vi "Main.vi"() -> ()   [LabVIEW 2019]
uses:
  <vilib>/Native 3D Graph/xcontrol/3DPC_SurfacePlot.xctl
  <vilib>/Analysis/coordinate.llb/3D Coordinate Conversion (Array).vi
  <vilib>/Analysis/_algsub.llb/Real Vector Norm.vi
  <vilib>/Utility/file.llb/Read Delimited Spreadsheet (DBL).vi
  <vilib>/Analysis/polynomials.llb/Polynomial Roots (DBL).vi
  <vilib>/Analysis/NI_AALPro.lvlib
  <vilib>/Analysis/NI_AAL_Geometry.lvlib
panel:
  out "chegada":dbl[](array[numeric])
  out "partida":dbl[](array[numeric])
  out "Areas dos triangulos":dbl[](array[numeric])
  out "Primeiro":dbl[](array[numeric])
  out "Ultimo":dbl[](array[numeric])
  out "origem z":dbl
  out "origem y":dbl
  out "origem x":dbl
  out "Roots YZ":cdb[](array[numeric])
  out "Roots XZ":cdb[](array[numeric])
  out "3D Graph 2":refnum<class "Base Datatype.lvclass">[](xcontrol)
  out "Right 2":cluster{"Y":dbl[], "Y":dbl[]}[](graph)
  out "Front 2":cluster{"Y":dbl[], "Y":dbl[]}[](graph)
  out "Top 2":cluster{"Y":dbl[], "Y":dbl[]}[](graph)
  out "Right":cluster{"Y":dbl[], "Y":dbl[]}[](graph)
  out "Front":cluster{"Y":dbl[], "Y":dbl[]}[](graph)
  out "Top":cluster{"Y":dbl[], "Y":dbl[]}[](graph)
  out "3D Graph":refnum<class "Base Datatype.lvclass">[](xcontrol)
  # "Localizaçao da origem"
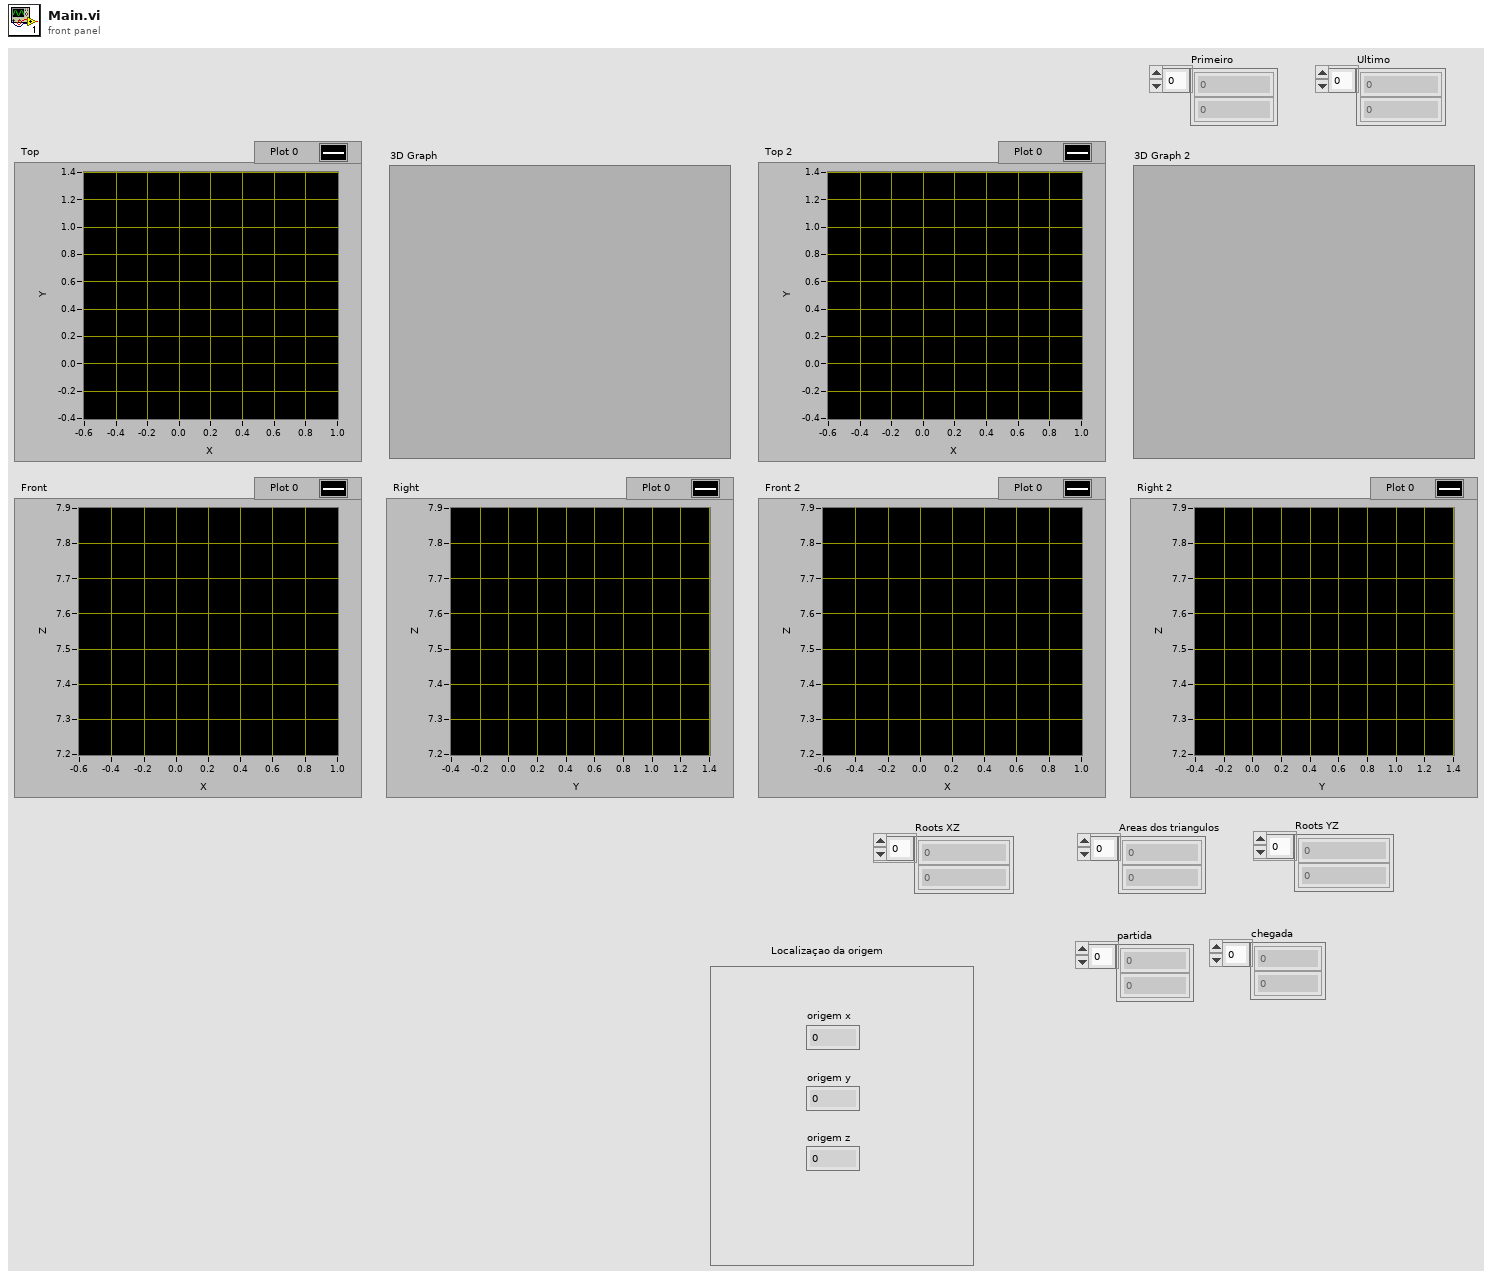
[diagram p1: front panel]
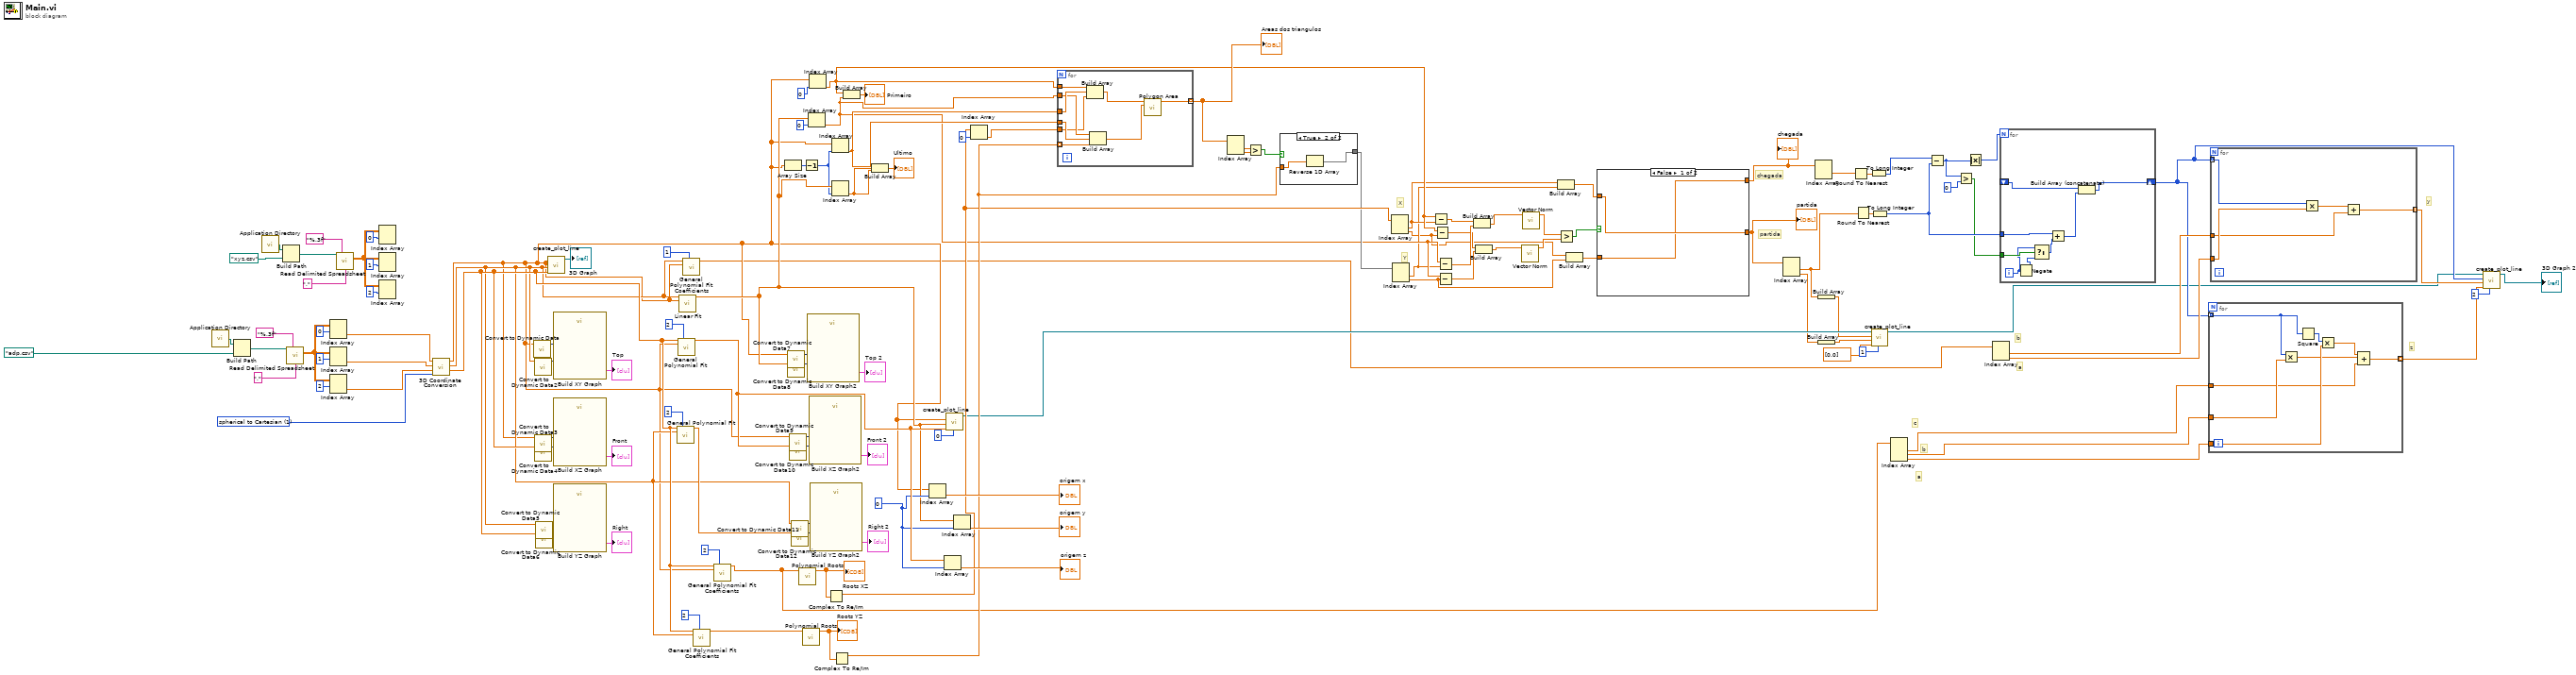
[diagram p0: block diagram]
diagram:
  w73 = 0
  w91 = u16 1 items=["Cartesian to spherical", "spherical to Cartesian", "Cartesian to cylindrical", "cylindrical to Cartesian", "spherical to cylindrical", "cylindrical to spherical"] ("conversion type")
  # "y"
  # "z"
  # "b"
  # "a"
  # "c"
  # "b"
  # "a"
  # "partida"
  # "chegada"
  # "Y"
  # "X"
  n1 = call <vilib>:"Application Directory.vi"() -> ("Application Directory"=w88:path)
  n2 = Build Path(base path=w88, name or relative path=path "adp.csv" ("file path (dialog if empty)")) -> (appended path=w89:path)
  n3 = call <vilib>:"Application Directory.vi"() -> ("Application Directory"=w123:path)
  n4 = Build Path(base path=w123, name or relative path=path "xyz.csv" ("file path (dialog if empty)")) -> (appended path=w124:path)
  n5 = call-poly <vilib>:"Read Delimited Spreadsheet.vi"("file path (dialog if empty)"=w89, "format (%.3f)"="%.3f", "delimiter (\\t)"="," ("delimiter (\\t)")) -> ("all rows"=w82:dbl[][])  [unwired: 7 in, 5 out]
  n6 = Index Array(array=w82, index (row)=0) -> (element=w78:dbl[])  [unwired: 1 in]
  n7 = Index Array(array=w82, index (row)=1) -> (element=w79:dbl[])  [unwired: 1 in]
  n8 = Index Array(array=w82, index (row)=2) -> (element=w80:dbl[])  [unwired: 1 in]
  n9 = call-poly <vilib>:"Read Delimited Spreadsheet.vi"("file path (dialog if empty)"=w124, "format (%.3f)"="%.3f", "delimiter (\\t)"="," ("delimiter (\\t)")) -> ("all rows"=w116:dbl[][])  [unwired: 7 in, 5 out]
  n10 = Index Array(array=w116, index (row)=0) -> ()  [unwired: 1 in, 1 out]
  n11 = Index Array(array=w116, index (row)=1) -> ()  [unwired: 1 in, 1 out]
  n12 = Index Array(array=w116, index (row)=2) -> ()  [unwired: 1 in, 1 out]
  n13 = call-poly <vilib>:"3D Coordinate Conversion.vi"("conversion type"=w91, "Axis 3"=w80, "Axis 2"=w79, "Axis 1"=w78) -> ("Axis 3 Out"=w81:dbl[], "Axis 2 Out"=w14:dbl[], "Axis 1 Out"=w13:dbl[])  [unwired: 4 in, 1 out]
  n14 = call "Convert to Dynamic Data"("Array"=w13) -> ("Dynamic Data Type"=w114:dynamicdata)  [unwired: 3 in]
  n15 = call "Convert to Dynamic Data2"("Array"=w14) -> ("Dynamic Data Type"=w113:dynamicdata)  [unwired: 3 in]
  n16 = call "Convert to Dynamic Data3"("Array"=w13) -> ("Dynamic Data Type"=w110:dynamicdata)  [unwired: 3 in]
  n17 = call "Convert to Dynamic Data4"("Array"=w81) -> ("Dynamic Data Type"=w109:dynamicdata)  [unwired: 3 in]
  n18 = call "Convert to Dynamic Data5"("Array"=w14) -> ("Dynamic Data Type"=w108:dynamicdata)  [unwired: 3 in]
  n19 = call "Convert to Dynamic Data6"("Array"=w81) -> ("Dynamic Data Type"=w107:dynamicdata)  [unwired: 3 in]
  n20 = call <vilib>:"create_plot_line.vi"("z vector"=w81, "y vector"=w14, "x vector"=w13) -> ("plots out"=→"3D Graph":refnum<class "Base Datatype.lvclass">[])  [unwired: 2 in, 6 out]
  n21 = call "Build XY Graph"("Y Input"=w113, "X Input"=w114) -> ("XY Graph"=→"Top":cluster{"X":dbl[], "Y":dbl[]}[])  [unwired: 8 in, 1 out]
  n22 = call "Build XZ Graph"("Y Input"=w109, "X Input"=w110) -> ("XY Graph"=→"Front":cluster{"X":dbl[], "Y":dbl[]}[])  [unwired: 8 in, 1 out]
  n23 = call "Build YZ Graph"("Y Input"=w107, "X Input"=w108) -> ("XY Graph"=→"Right":cluster{"X":dbl[], "Y":dbl[]}[])  [unwired: 8 in, 1 out]
  n24 = call <vilib>:"General Polynomial Fit.vi"("Y"=w81, "polynomial order"=2, "X"=w14) -> ("Best Polynomial Fit"=w95:dbl[])  [unwired: 9 in, 3 out]
  n25 = call <vilib>:"General Polynomial Fit.vi"("Y"=w81, "polynomial order"=2, "X"=w13) -> ("Best Polynomial Fit"=w75:dbl[])  [unwired: 9 in, 3 out]
  n26 = call <vilib>:"Linear Fit.vi"("Y"=w14, "X"=w13) -> ("Best Linear Fit"=w70:dbl[])  [unwired: 9 in, 4 out]
  n27 = call <vilib>:"General Polynomial Fit Coefficients.vi"("Y"=w14, "polynomial order"=1, "X"=w13) -> ("Polynomial Coefficients"=w11:dbl[])  [unwired: 11 in, 1 out]
  n28 = call <vilib>:"General Polynomial Fit Coefficients.vi"("Y"=w81, "polynomial order"=2, "X"=w14) -> ("Polynomial Coefficients"=w92:dbl[])  [unwired: 11 in, 1 out]
  n29 = call <vilib>:"General Polynomial Fit Coefficients.vi"("Y"=w81, "polynomial order"=2, "X"=w13) -> ("Polynomial Coefficients"=w32:dbl[])  [unwired: 11 in, 1 out]
  n30 = Array Size(array=w13) -> (size(s)=w67:i32)
  n31 = call "Convert to Dynamic Data7"("Array"=w13) -> ("Dynamic Data Type"=w105:dynamicdata)  [unwired: 3 in]
  n32 = call "Convert to Dynamic Data8"("Array"=w70) -> ("Dynamic Data Type"=w106:dynamicdata)  [unwired: 3 in]
  n33 = call "Convert to Dynamic Data9"("Array"=w13) -> ("Dynamic Data Type"=w102:dynamicdata)  [unwired: 3 in]
  n34 = call "Convert to Dynamic Data10"("Array"=w75) -> ("Dynamic Data Type"=w103:dynamicdata)  [unwired: 3 in]
  n35 = call "Convert to Dynamic Data11"("Array"=w14) -> ("Dynamic Data Type"=w99:dynamicdata)  [unwired: 3 in]
  n36 = call "Convert to Dynamic Data12"("Array"=w95) -> ("Dynamic Data Type"=w100:dynamicdata)  [unwired: 3 in]
  n37 = call-poly <vilib>:"Polynomial Roots.vi"("P(x)"=w32) -> ("Roots"=w65:cdb[])  [unwired: 9 in, 1 out]
  "Roots XZ" <- w65
  n38 = call-poly <vilib>:"Polynomial Roots.vi"("P(x)"=w92) -> ("Roots"=w64:cdb[])  [unwired: 9 in, 1 out]
  "Roots YZ" <- w64
  n39 = Decrement(x=w67) -> (x-1=w66:i32)
  n40 = call "Build XY Graph2"("Y Input"=w106, "X Input"=w105) -> ("XY Graph"=→"Top 2":cluster{"X":dbl[], "Y":dbl[]}[])  [unwired: 8 in, 1 out]
  n41 = Index Array(array=w70, index=0) -> (element=w51:dbl)
  n42 = Index Array(array=w13, index=0) -> (element=w52:dbl)
  n43 = call "Build XZ Graph2"("Y Input"=w103, "X Input"=w102) -> ("XY Graph"=→"Front 2":cluster{"X":dbl[], "Y":dbl[]}[])  [unwired: 8 in, 1 out]
  n44 = call "Build YZ Graph2"("Y Input"=w100, "X Input"=w99) -> ("XY Graph"=→"Right 2":cluster{"X":dbl[], "Y":dbl[]}[])  [unwired: 8 in, 1 out]
  n45 = Complex To Re/Im(x + iy=w65) -> (x=w54:dbl[])  [unwired: 1 out]
  n46 = Index Array(array=w13, index=w66) -> (element=w63:dbl)
  n47 = Index Array(array=w70, index=w66) -> (element=w62:dbl)
  n48 = Complex To Re/Im(x + iy=w64) -> (x=w55:dbl[])  [unwired: 1 out]
  n49 = Build Array(w52, w51) -> (→"Primeiro":dbl[])
  n50 = Build Array(w63, w62) -> (→"Ultimo":dbl[])
  n51 = Index Array(array=w13, index=w73) -> (element=→"origem x":dbl)
  n52 = Index Array(array=w75, index=w73) -> (element=→"origem z":dbl)
  n53 = call <vilib>:"create_plot_line.vi"("plot ID"=0, "z vector"=w75, "y vector"=w70, "x vector"=w13) -> ("plots out"=w37:refnum<class "Base Datatype.lvclass">[])  [unwired: 1 in, 6 out]
  n54 = Index Array(array=w70, index=w73) -> (element=→"origem y":dbl)
  n55 = Index Array(array=w54, index=0) -> (element=w60:dbl)
  n56 = for {
    tunnel: w55 -> [w130] mode=indexing
    tunnel: w52 -> [w134]
    tunnel: w51 -> [w132]
    tunnel: w63 -> [w133]
    tunnel: w62 -> [w131]
    tunnel: [w127] -> w59 mode=indexing
    tunnel: w60 -> [w126]
    n57 = Build Array(w134, w133, w126) -> (w128:dbl[])
    n58 = Build Array(w132, w131, w130) -> (w129:dbl[])
    n59 = call <vilib>:"Polygon Area.vi"("Y"=w129, "X"=w128) -> ("signed area"=w127:dbl)  [unwired: 8 in, 1 out]
  }
  "Areas dos triangulos" <- w59
  n60 = Index Array(array=w59) -> (element #1=w57:dbl, element #2=w58:dbl)  [unwired: 2 in]
  n61 = Greater?(x=w57, y=w58) -> (0:w56:bool)
  n62 = case shown="True" w56 {
    tunnel: w55 -> [w135 w137]
    tunnel: [w135 w136] -> w53
    frame False {
    }
    frame True {
      n63 = Reverse 1D Array(array=w137) -> (reversed array=w136:dbl[])
    }
  }
  n64 = Index Array(array=w54) -> (element #1=w41:dbl, element #2=w39:dbl)  [unwired: 2 in]
  n65 = Index Array(array=w53) -> (element #1=w40:dbl, element #2=w38:dbl)  [unwired: 2 in]
  n66 = Subtract(x=w52, y=w41) -> (x-y=w50:dbl)
  n67 = Subtract(x=w52, y=w39) -> (x-y=w48:dbl)
  n68 = Subtract(x=w51, y=w40) -> (x-y=w49:dbl)
  n69 = Subtract(x=w51, y=w38) -> (x-y=w47:dbl)
  n70 = Build Array(w50, w49) -> (w43:dbl[])
  n71 = Build Array(w48, w47) -> (w42:dbl[])
  n72 = call-poly <vilib>:"Vector Norm.vi"("Input Vector"=w42) -> ("norm"=w45:dbl)  [unwired: 9 in, 1 out]
  n73 = call-poly <vilib>:"Vector Norm.vi"("Input Vector"=w43) -> ("norm"=w46:dbl)  [unwired: 9 in, 1 out]
  n74 = Build Array(w41, w40) -> (w30:dbl[])
  n75 = Greater?(x=w46, y=w45) -> (0:w44:bool)
  n76 = Build Array(w39, w38) -> (w31:dbl[])
  n77 = case shown="False" w44 {
    tunnel: [w139 w141] -> w29
    tunnel: w31 -> [w138 w141]
    tunnel: w30 -> [w139 w140]
    tunnel: [w138 w140] -> w28
    frame False {
    }
    frame True {
    }
  }
  "partida" <- w29
  "chegada" <- w28
  n78 = Index Array(array=w29) -> (element #1=w26:dbl, element #2=w35:dbl)  [unwired: 2 in]
  n79 = Index Array(array=w28) -> (element #1=w27:dbl)  [unwired: 2 in, 1 out]
  n80 = Build Array(w26) -> (w36:dbl[])
  n81 = Build Array(w35) -> (w34:dbl[])
  n82 = Round To Nearest(number=w27) -> (nearest integer value=w25:dbl)
  n83 = Round To Nearest(number=w26) -> (nearest integer value=w24:dbl)
  n84 = To Long Integer(number=w25) -> (32bit integer=w23:i32)
  n85 = call <vilib>:"create_plot_line.vi"("plot ID"=1, "z vector"=dbl[] [0.0], "y vector"=w34, "x vector"=w36, "plots in"=w37) -> ("plots out"=w5:refnum<class "Base Datatype.lvclass">[])  [unwired: 6 out]
  n86 = To Long Integer(number=w24) -> (32bit integer=w22:i32)
  n87 = Index Array(array=w32) -> (element #1=w15:dbl, element #2=w16:dbl, element #3=w17:dbl)  [unwired: 3 in]
  n88 = Subtract(x=w23, y=w22) -> (x-y=w18:i32)
  n89 = Greater?(x=w18, y=0) -> (0:w19:bool)
  n90 = Absolute Value(x=w18) -> (abs(x)=w21:i32)
  n91 = Index Array(array=w11) -> (element #1=w9:dbl, element #2=w10:dbl)  [unwired: 2 in]
  n92 = for {
    N: w21 -> [_]
    shift-right: [w146] -> w6
    shift-left: _ -> [w149]
    tunnel: w22 -> [w148]
    tunnel: w19 -> [w145]
    i -> [w143]
    n93 = Negate(x=w143) -> (-x=w144:i32)
    n94 = Select(t=w143, s=w145, f=w144) -> (s? t:f=w142:i32)
    n95 = Add(x=w148, y=w142) -> (x+y=w147:i32)
    n96 = Build Array (concatenate)(w149, w147) -> (w146:i32[])
  }
  n97 = for {
    tunnel: w17 -> [w156]
    tunnel: w16 -> [w154]
    tunnel: w15 -> [w151]
    tunnel: w6 -> [w155] mode=indexing
    tunnel: [w150] -> w8 mode=indexing
    n98 = Multiply(x=w155, y=w154) -> (x*y=w152:dbl)
    n99 = Square(x=w155) -> (x^2=w157:i32)
    n100 = Multiply(x=w157, y=w156) -> (x*y=w153:dbl)
    n101 = Compound Arithmetic op=ADD(w153, w152, w151) -> (w150:dbl)
  }
  n102 = for {
    tunnel: w6 -> [w161] mode=indexing
    tunnel: w10 -> [w162]
    tunnel: w9 -> [w160]
    tunnel: [w158] -> w7 mode=indexing
    n103 = Multiply(x=w161, y=w162) -> (x*y=w159:dbl)
    n104 = Add(x=w159, y=w160) -> (x+y=w158:dbl)
  }
  n105 = call <vilib>:"create_plot_line.vi"("plot ID"=2, "z vector"=w8, "y vector"=w7, "x vector"=w6, "plots in"=w5) -> ("plots out"=→"3D Graph 2":refnum<class "Base Datatype.lvclass">[])  [unwired: 6 out]
